vi "Messwerte schreiben.vi"(0 "VISA resource name":refnum<visa-resource-name>, 1 "path":path) -> (2 "VISA resource name 2":refnum<visa-resource-name>, 3 "File Refnumber":path, 4 "path 2":path)   [LabVIEW 2021]
uses:
  Global Variabeln.vi
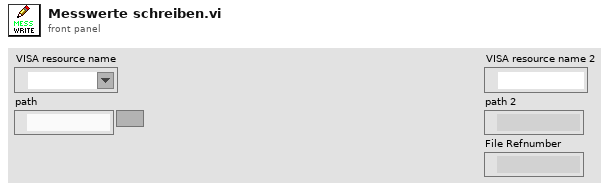
[diagram p1: front panel]
types:
  T1 = enum16{"open", "replace", "create", "open or create", "replace or create", "replace or create with confirmation"}
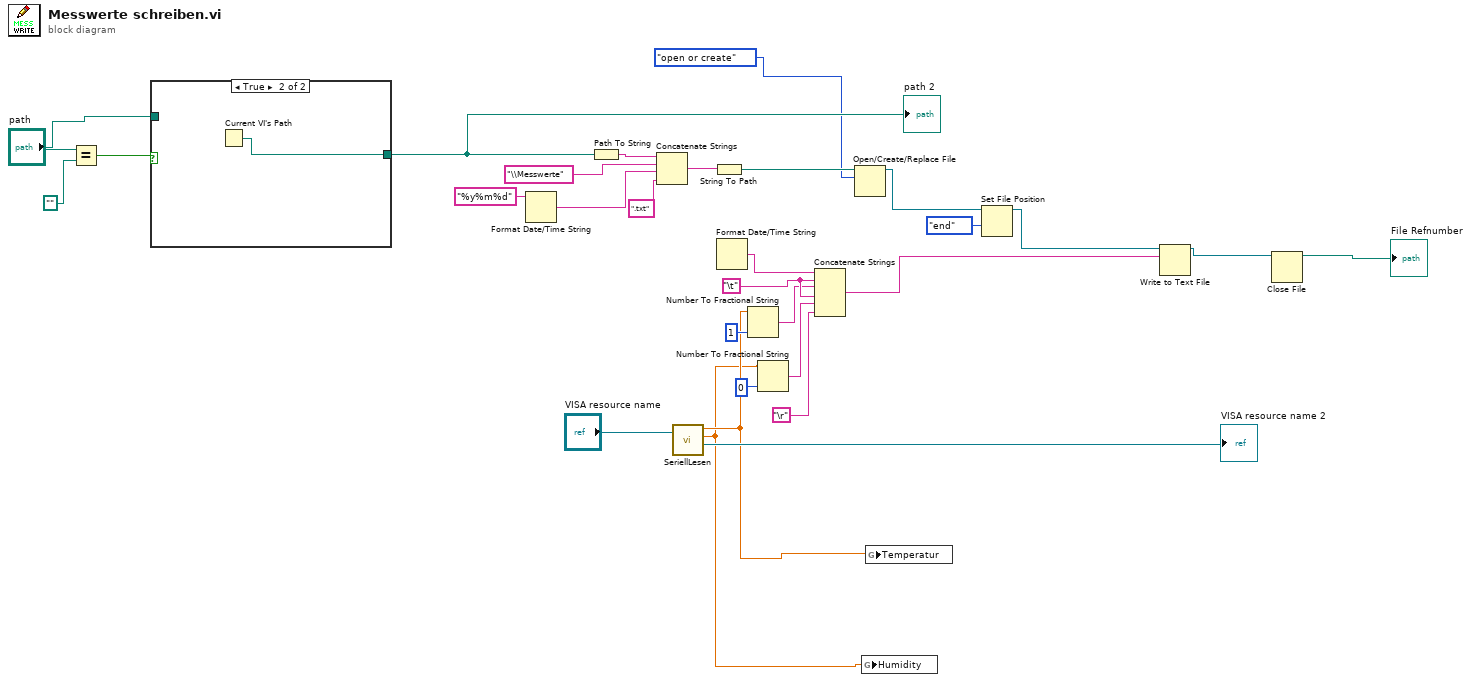
[diagram p0: block diagram]
diagram:
  w27 = "\t"
  n1 = Equal?(x="path", y=path "") -> (x = y?=w7:bool)
  n2 = case shown="True" w7 {
    tunnel: [w30 w31] -> w5
    tunnel: "path" -> [w30 _]
    frame False {
    }
    frame True {
      n3 = Current VI's Path() -> (path=w31:path)
    }
  }
  "path 2" <- w5
  n4 = Format Date/Time String(time format string (%c)="%y%m%d") -> (date/time string=w11:string)  [unwired: 2 in]
  n5 = Path To String(path=w5) -> (string=w16:string)
  n6 = Concatenate Strings(w16, "\\Messwerte" ("string"), w11, ".txt" ("string")) -> (w15:string)
  n7 = call "SeriellLesen.vi"("VISA resource name"="VISA resource name") -> ("Temperatur"=w3:dbl, "Humidity"=w2:dbl, "VISA resource name 2"=→"VISA resource name 2":refnum<visa-resource-name>)  [unwired: 1 in, 1 out]
  n8 = String To Path(string=w15) -> (path=w14:path)
  n9 = Format Date/Time String() -> (date/time string=w28:string)  [unwired: 3 in]
  n10 = Number To Fractional String(number=w3, precision (6)=i16 1) -> (F-format string=w18:string)  [unwired: 2 in]
  n11 = Number To Fractional String(number=w2, precision (6)=i16 0) -> (F-format string=w20:string)  [unwired: 2 in]
  n12 = Concatenate Strings(w28, w27, w18, w27, w20, "\r") -> (w25:string)
  n13 = Open/Create/Replace File(file path (use dialog)=w14, operation (0:open)=T1."open or create") -> (refnum out=w24:refnum<file>)  [unwired: 4 in, 2 out]
  n14 = global write "Global Variabeln.vi" "Humidity"(w2) -> ()
  n15 = global write "Global Variabeln.vi" "Temperatur"(w3) -> ()
  n16 = Set File Position(refnum=w24, from (0:start)=enum16{"start", "end", "current"}."end") -> (refnum out=w23:refnum<file>)  [unwired: 2 in, 1 out]
  n17 = Write to Text File(file (use dialog)=w23, text=w25) -> (refnum out=w21:refnum<file>)  [unwired: 2 in, 2 out]
  n18 = Close File(refnum=w21) -> (path=→"File Refnumber":path)  [unwired: 1 in, 1 out]
